vi "Updater Convert TDMS Test Runs 4.3 to 5.0 S Parameter.vi"(7 "Source TDMS File In":refnum<k34>, 8 "error in (no error)":errorcluster, 10 "Group Name In":string, 11 "New TDMS File In":refnum<k34>) -> (0 "error out":errorcluster, 2 "Group Name Out":string, 3 "New TDMS File Out":refnum<k34>, 5 "Source TDMS File Out":refnum<k34>)   [LabVIEW 2011]
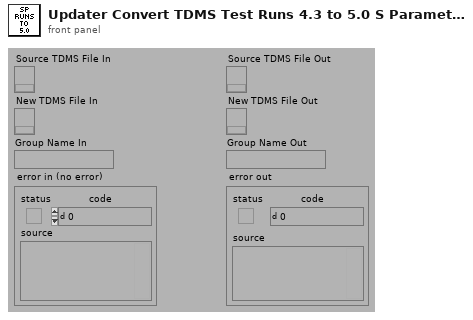
[diagram p1: front panel]
types:
  T1 = typedef "SP Channel Type.ctl" = enum16{"Frequency", "Data", "Limit", "Adapter", "Memory", "Value", "Value Limit"}
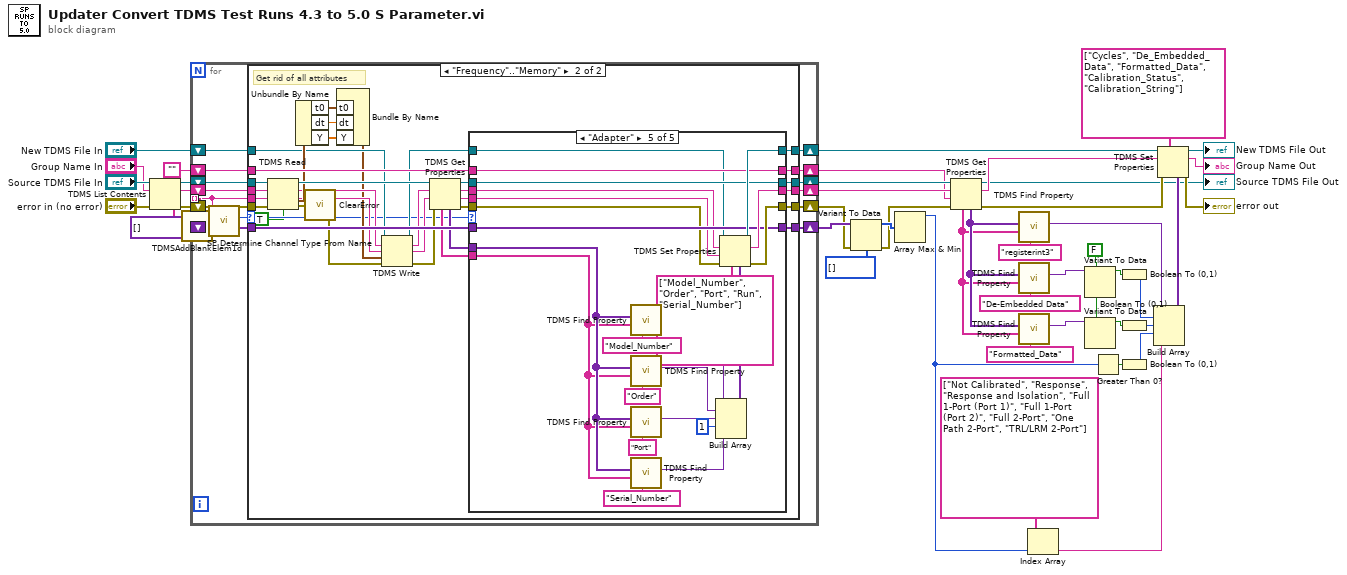
[diagram p0: block diagram]
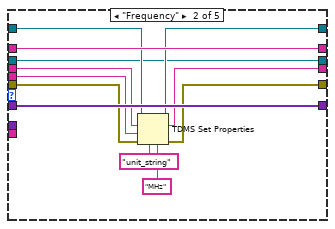
[diagram p4: hidden frame]
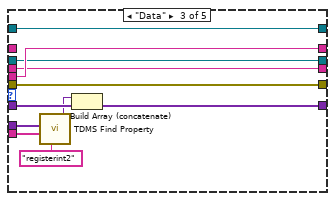
[diagram p5: hidden frame]
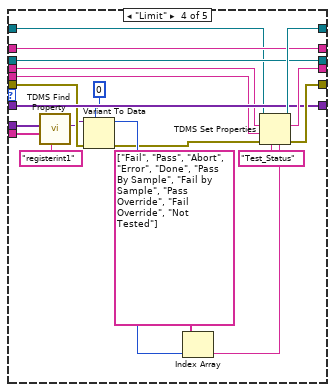
[diagram p6: hidden frame]
diagram:
  w2 = FALSE
  n1 = TDMS List Contents(4:"error in (no error)", 6:"Group Name In", 7:"Source TDMS File In") -> (0:w43:errorcluster, 1:w1:string[], 2:w41:string, 3:w42:refnum<k34>)
  n2 = call <vilib>:"TDMSAddBlankElem1d.vi"("input string array"=w1) -> ("output string array with blank element at the beginning"=w40:string[])
  n3 = for {
    shift-right: [w59] -> w18
    shift-left: w43 -> [w52]
    shift-right: [w60] -> w38
    shift-left: w42 -> [w51]
    tunnel: w40 -> [w49] mode=indexing
    shift-right: [w54] -> w37
    shift-left: w41 -> [w50]
    shift-right: [w58] -> w19
    shift-left: "" -> [w57]
    shift-right: [w55] -> w22
    shift-left: variant[] [] -> [w56]
    shift-right: [w53] -> w24
    shift-left: "New TDMS File In" -> [w48]
    n4 = call "SP Determine Channel Type From Name.vi"("Channel Name"=w49) -> ("Channel Type"=w47:T1)  [unwired: 10 out]
    n5 = case shown="\"Frequency\"..\"Memory\"" w47 {
      selector: w47 -> [_ w69]
      tunnel: [w66 w101] -> w60
      tunnel: [w62 w100] -> w59
      tunnel: [w64 w99] -> w58
      tunnel: w57 -> [w64 w98]
      tunnel: w56 -> [w61 w97]
      tunnel: [w61 w96] -> w55
      tunnel: [w65 w95] -> w54
      tunnel: [w63 w94] -> w53
      tunnel: w52 -> [w62 w89]
      tunnel: w51 -> [w66 w87]
      tunnel: w50 -> [w65 w86]
      tunnel: w49 -> [_ w85]
      tunnel: w48 -> [w63 w78]
      frame Default {
        # "Empty channel for Group level."
      }
      frame "Frequency".."Memory" {
        # "Get rid of all attributes"
        n6 = TDMS Read(0:w87, 5:w86, 7:w85, 11:w89, 13:TRUE ("return channels in file order? (F)")) -> (4:w88:refnum<k34>, 6:w76:string, 8:w75:string, 10:w84:waveform(dbl), 15:w68:errorcluster)  [unwired: 3 in, 1 out]
        n7 = Unbundle By Name(w84) -> ("t0"=w83:timestamp, "dt"=w82:dbl, "Y"=w81:dbl[])
        n8 = call <vilib>:"ClearError.vi"("error in (no error)"=w68) -> ("error out"=w77:errorcluster)
        n9 = Bundle By Name("t0"=w83, "dt"=w82, "Y"=w81) -> (w70:waveform(dbl))  [unwired: 1 out]
        n10 = TDMS Write(0:w78, 5:w76, 7:w75, 9:w70, 11:w77) -> (4:w71:refnum<k34>, 6:w73:string, 8:w74:string, 15:w72:errorcluster)  [unwired: 1 in]
        n11 = TDMS Get Properties(8:w72, 9:w74, 10:w73, 11:w88) -> (0:w93:errorcluster, 1:w92:string, 2:w91:string, 3:w90:refnum<k34>, 4:w79:variant[], 6:w80:string[])  [unwired: 2 out]
        n12 = case shown="\"Adapter\"" w69 {
          tunnel: w93 -> [w106 w108 w120 w138 w151]
          tunnel: w91 -> [w103 w110 w122 w132 w153]
          tunnel: w90 -> [w107 w111 w124 w139 w165]
          tunnel: [w107 w111 w124 w139 w165] -> w101
          tunnel: [w106 w116 w120 w148 w171] -> w100
          tunnel: w92 -> [_ w109 w125 w133 w152]
          tunnel: [w105 w119 w125 w147 w170] -> w99
          tunnel: w98 -> [w105 w119 _ w147 w170]
          tunnel: w97 -> [w104 w118 w130 w146 w169]
          tunnel: [w104 w118 w129 w146 w169] -> w96
          tunnel: [w103 w115 w122 w149 w172] -> w95
          tunnel: w71 -> [w102 w112 w121 w131 w154]
          tunnel: [w102 w117 w121 w150 w173] -> w94
          tunnel: w80 -> [_ _ w127 w140 w155]
          tunnel: w79 -> [_ _ w128 w141 w156]
          frame "Memory", Default {
          }
          frame "Frequency" {
            n13 = TDMS Set Properties(5:"MHz", 7:"unit_string", 8:w108, 9:w109, 10:w110, 11:w112) -> (0:w116:errorcluster, 2:w115:string, 3:w117:refnum<k34>)  [unwired: 1 out]
          }
          frame "Data" {
            n14 = call "TDMS Find Property.vi"("Property Name"="registerint2", "Property Names"=w127, "Property Values"=w128) -> ("Property Value"=w123:variant)  [unwired: 5 out]
            n15 = Build Array (concatenate)(w123, w130) -> (w129:variant[])
          }
          frame "Limit" {
            n16 = call "TDMS Find Property.vi"("Property Name"="registerint1", "Property Names"=w140, "Property Values"=w141) -> ("Property Value"=w136:variant)  [unwired: 5 out]
            n17 = Variant To Data(error in=w138, type=0, Variant=w136) -> (data=w135:i32, error out=w134:errorcluster)
            n18 = Index Array(array=string[] ["Fail", "Pass", "Abort", "Error", "Done", "Pass By Sample", "Fail by Sample", "Pass Override", "Fail Override", "Not Tested"], index=w135) -> (element=w144:string)
            n19 = TDMS Set Properties(5:w144, 7:"Test_Status", 8:w134, 9:w133, 10:w132, 11:w131) -> (0:w148:errorcluster, 2:w149:string, 3:w150:refnum<k34>)  [unwired: 1 out]
          }
          frame "Adapter" {
            n20 = call "TDMS Find Property.vi"("Property Name"="Model_Number", "Property Names"=w155, "Property Values"=w156) -> ("Property Value"=w160:variant)  [unwired: 5 out]
            n21 = call "TDMS Find Property.vi"("Property Name"="Order", "Property Names"=w155, "Property Values"=w156) -> ("Property Value"=w159:variant)  [unwired: 5 out]
            n22 = call "TDMS Find Property.vi"("Property Name"="Port", "Property Names"=w155, "Property Values"=w156) -> ("Property Value"=w158:variant)  [unwired: 5 out]
            n23 = call "TDMS Find Property.vi"("Property Name"="Serial_Number", "Property Names"=w155, "Property Values"=w156) -> ("Property Value"=w157:variant)  [unwired: 5 out]
            n24 = Build Array(w160, w159, w158, 1, w157) -> (w166:variant[])
            n25 = TDMS Set Properties(5:w166, 7:string[] ["Model_Number", "Order", "Port", "Run", "Serial_Number"], 8:w151, 9:w152, 10:w153, 11:w154) -> (0:w171:errorcluster, 2:w172:string, 3:w173:refnum<k34>)  [unwired: 1 out]
          }
        }
      }
    }
  }
  n26 = Variant To Data(error in=w18, type=i32[] [], Variant=w22) -> (data=w20:i32[], error out=w17:errorcluster)
  n27 = Array Max & Min(array=w20) -> (max value=w33:i32)  [unwired: 3 out]
  n28 = TDMS Get Properties(8:w17, 9:w19, 10:w37, 11:w38) -> (0:w35:errorcluster, 2:w31:string, 3:→"Source TDMS File Out":refnum<k34>, 4:w13:variant[], 6:w12:string[])  [unwired: 1 in, 2 out]
  n29 = call "TDMS Find Property.vi"("Property Name"="registerint3", "Property Names"=w12, "Property Values"=w13) -> ("Property Value"=w11:variant)  [unwired: 5 out]
  n30 = call "TDMS Find Property.vi"("Property Name"="De-Embedded Data", "Property Names"=w12, "Property Values"=w13) -> ("Property Value"=w10:variant)  [unwired: 5 out]
  n31 = call "TDMS Find Property.vi"("Property Name"="Formatted_Data", "Property Names"=w12, "Property Values"=w13) -> ("Property Value"=w9:variant)  [unwired: 5 out]
  n32 = Index Array(array=string[] ["Not Calibrated", "Response", "Response and Isolation", "Full 1-Port (Port 1)", "Full 1-Port (Port 2)", "Full 2-Port", "One Path 2-Port", "TRL/LRM 2-Port"], index=w33) -> (element=w27:string)
  n33 = Variant To Data(type=w2, Variant=w10) -> (data=w8:bool)  [unwired: 1 in, 1 out]
  n34 = Variant To Data(type=w2, Variant=w9) -> (data=w6:bool)  [unwired: 1 in, 1 out]
  n35 = Greater Than 0?(x=w33) -> (x > 0?=w4:bool)
  n36 = Boolean To (0,1)(Boolean=w8) -> (0, 1=w7:i16)
  n37 = Boolean To (0,1)(Boolean=w6) -> (0, 1=w5:i16)
  n38 = Boolean To (0,1)(Boolean=w4) -> (0, 1=w3:i16)
  n39 = Build Array(w11, w7, w5, w3, w27) -> (w32:variant[])
  n40 = TDMS Set Properties(5:w32, 7:string[] ["Cycles", "De_Embedded_Data", "Formatted_Data", "Calibration_Status", "Calibration_String"], 8:w35, 10:w31, 11:w24) -> (0:→"error out":errorcluster, 2:→"Group Name Out":string, 3:→"New TDMS File Out":refnum<k34>)  [unwired: 2 out]
